vi "Init Agilent Channels Wilt.vi"(0 "Agilent Number":i32, 1 "VISA Resource Name":refnum<visa-resource-name>, 5 "Agilent Channels Array":T1[](array[typedef]), 11 "error in (no error)":errorcluster) -> (4 "Number of Read Channels":i32, 15 "error out":errorcluster)   [LabVIEW 2012]
uses:
  Agilent Channel Definition.ctl
  Drivers/Agilent 34970/Agilent 34970.lvlib
panel:
  out "Channel List":string
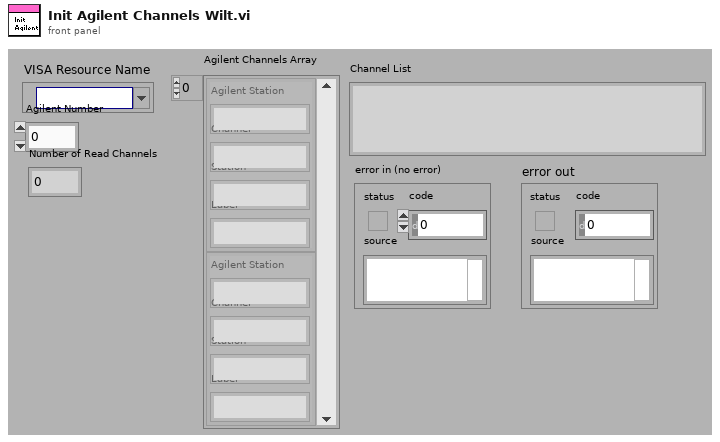
[diagram p1: front panel]
types:
  T1 = typedef "Agilent Channel Definition.ctl" = cluster{"Channel":string, "Station":string, "Label":string, "Agilent Station":string}
  T2 = cluster{"Thermocouple Type (Last)":enum16{"B", "E", "J", "K", "N", "R", "S", "T", "Default (Last)"}, "TC Rjunction (2:Int)":enum16{"Fixed", "External", "Internal"}, "Fixed Rjunction Temp (0:Manual)":enum16{"Manual", "Minimum", "Maximum"}, "TC Auto Check? (F:Don't Check)":bool, "Rjunct Temp Value (0)":dbl}
  T3 = enum16{"100 mV", "1 V", "10 V", "100 V", "300 V", "Minimum", "Maximum"}
  T4 = enum16{"100 Ohm", "1 kOhm", "10 kOhm", "100 kOhm", "1 MOhm", "10 MOhm", "100 MOhm", "Minimum", "Maximum"}
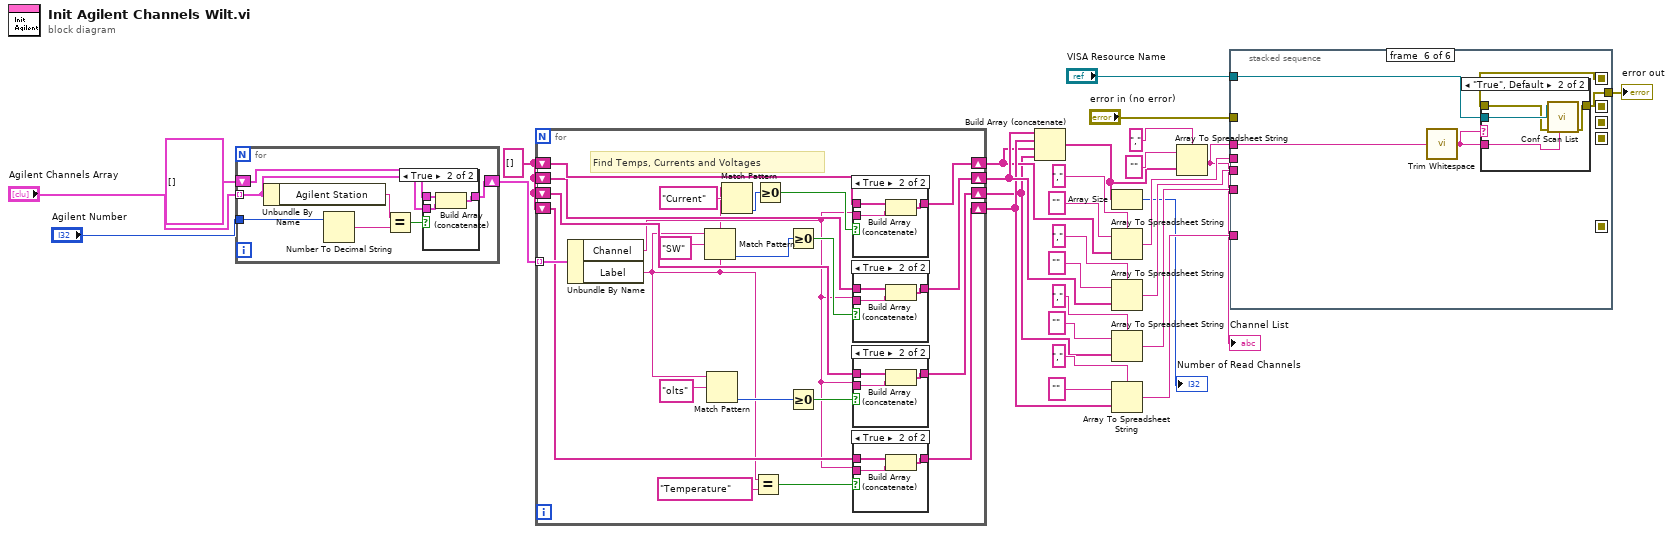
[diagram p0: block diagram]
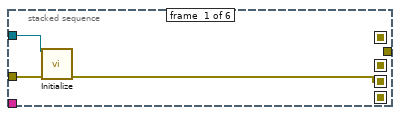
[diagram p3: hidden frame]
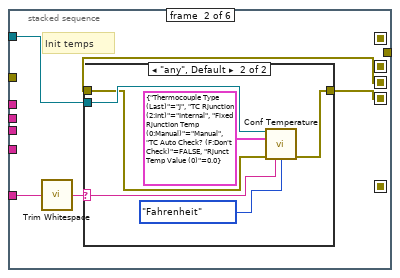
[diagram p4: hidden frame]
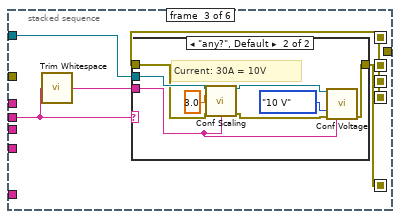
[diagram p6: hidden frame]
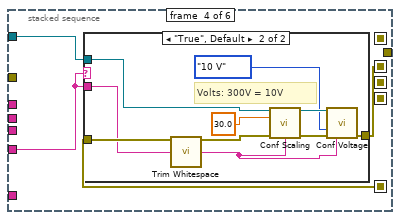
[diagram p8: hidden frame]
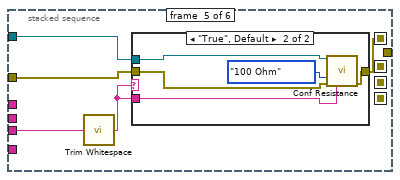
[diagram p10: hidden frame]
diagram:
  w13 = string[] []
  n1 = for {
    tunnel: "Agilent Channels Array" -> [w34] mode=indexing
    tunnel: "Agilent Number" -> [w31]
    shift-right: [w33] -> w14
    shift-left: T1[] [] -> [w32]
    n2 = Unbundle By Name(w34) -> ("Agilent Station"=w35:string)
    n3 = Number To Decimal String(number=w31) -> (decimal integer string=w36:string)  [unwired: 1 in]
    n4 = Equal?(x=w35, y=w36) -> (x = y?=w30:bool)
    n5 = case shown="True" w30 {
      tunnel: w34 -> [_ w40]
      tunnel: [w37 w39] -> w33
      tunnel: w32 -> [w37 w38]
      frame False {
      }
      frame True {
        n6 = Build Array (concatenate)(w38, w40) -> (w39:T1[])
      }
    }
  }
  n7 = for {
    tunnel: w14 -> [w62] mode=indexing
    shift-right: [w59] -> w6
    shift-left: w13 -> [w58]
    shift-right: [w54] -> w5
    shift-left: w13 -> [w53]
    shift-right: [w49] -> w4
    shift-left: w13 -> [w48]
    shift-right: [w44] -> w7
    shift-left: w13 -> [w43]
    # "Find Temps, Currents and Voltages"
    n8 = Unbundle By Name(w62) -> ("Channel"=w42:string, "Label"=w41:string)
    n9 = Match Pattern(string=w41, regular expression="SW") -> (offset past match=w46:i32)  [unwired: 1 in, 3 out]
    n10 = Match Pattern(string=w41, regular expression="olts") -> (offset past match=w51:i32)  [unwired: 1 in, 3 out]
    n11 = Match Pattern(string=w41, regular expression="Current") -> (offset past match=w56:i32)  [unwired: 1 in, 3 out]
    n12 = Equal?(x=w41, y="Temperature") -> (x = y?=w60:bool)
    n13 = Greater Or Equal To 0?(x=w56) -> (x >= 0?=w55:bool)
    n14 = Greater Or Equal To 0?(x=w46) -> (x >= 0?=w47:bool)
    n15 = Greater Or Equal To 0?(x=w51) -> (x >= 0?=w50:bool)
    n16 = case shown="True" w55 {
      tunnel: w42 -> [_ w74]
      tunnel: [w71 w73] -> w54
      tunnel: w53 -> [w71 w72]
      frame False {
      }
      frame True {
        n17 = Build Array (concatenate)(w72, w74) -> (w73:string[])
      }
    }
    n18 = case shown="True" w47 {
      tunnel: w42 -> [_ w66]
      tunnel: [w63 w65] -> w44
      tunnel: w43 -> [w63 w64]
      frame False {
      }
      frame True {
        n19 = Build Array (concatenate)(w64, w66) -> (w65:string[])
      }
    }
    n20 = case shown="True" w50 {
      tunnel: w42 -> [_ w70]
      tunnel: [w67 w69] -> w49
      tunnel: w48 -> [w67 w68]
      frame False {
      }
      frame True {
        n21 = Build Array (concatenate)(w68, w70) -> (w69:string[])
      }
    }
    n22 = case shown="True" w60 {
      tunnel: w42 -> [_ w78]
      tunnel: [w75 w77] -> w59
      tunnel: w58 -> [w75 w76]
      frame False {
      }
      frame True {
        n23 = Build Array (concatenate)(w76, w78) -> (w77:string[])
      }
    }
  }
  n24 = Build Array (concatenate)(w7, w6, w5, w4) -> (w2:string[])
  n25 = Array Size(array=w2) -> (size(s)=→"Number of Read Channels":i32)
  n26 = Array To Spreadsheet String(delimiter (Tab)=",", array=w5, 3:"" ("format string")) -> (spreadsheet string=w22:string)
  n27 = Array To Spreadsheet String(delimiter (Tab)=",", array=w7, 3:"" ("format string")) -> (spreadsheet string=w10:string)
  n28 = Array To Spreadsheet String(delimiter (Tab)=",", array=w4, 3:"" ("format string")) -> (spreadsheet string=w20:string)
  n29 = Array To Spreadsheet String(delimiter (Tab)=",", array=w6, 3:"" ("format string")) -> (spreadsheet string=w27:string)
  n30 = Array To Spreadsheet String(delimiter (Tab)=",", array=w2, 3:"" ("format string")) -> (spreadsheet string=w3:string)
  "Channel List" <- w3
  n31 = stacked-sequence {
    seq-local: [_ _ _ w109 _ _] -> [_ _ _ _ _ _]
    seq-local: [_ _ w96 _ _ _] -> [_ _ _ w110 _ _]
    seq-local: [_ w85 _ _ _ _] -> [_ _ w97 _ _ _]
    seq-local: [w80 _ _ _ _ _] -> [_ w84 _ _ _ _]
    seq-local: [_ _ _ _ w124 _] -> [_ _ _ _ _ w135]
    tunnel: w27 -> [_ w83 _ _ _ _]
    tunnel: "VISA Resource Name" -> [w79 w86 w98 w111 w125 w137]
    tunnel: w22 -> [_ _ w94 _ _ _]
    tunnel: w20 -> [_ _ _ w108 _ _]
    tunnel: "error in (no error)" -> [w81 _ _ _ w126 _]
    tunnel: [_ _ _ _ _ w136] -> w18
    tunnel: w10 -> [_ _ _ _ w123 _]
    tunnel: w3 -> [_ _ _ _ _ w134]
    frame #0 {
      n32 = call "Initialize.vi"("VISA Resource Name"=w79, "error in (no error)"=w81) -> ("error out"=w80:errorcluster)  [unwired: 12 in, 1 out]
    }
    frame #1 {
      # "Init temps"
      n33 = call <vilib>:"Trim Whitespace.vi"("string"=w83) -> ("trimmed string"=w82:string)  [unwired: 1 in]
      n34 = case shown="\"any\", Default" w82 {
        selector: w82 -> [_ w88]
        tunnel: w86 -> [_ w91]
        tunnel: [w87 w90] -> w85
        tunnel: w84 -> [w87 w89]
        frame "" {
        }
        frame "any", Default {
          n35 = call "Conf Temperature.vi"("VISA Resource Name"=w91, "Thermocouple Configuration"=T2 {"Thermocouple Type (Last)"=enum."J", "TC Rjunction (2:Int)"=enum."Internal", "Fixed Rjunction Temp (0:Manual)"=enum."Manual", "TC Auto Check? (F:Don't Check)"=FALSE, "Rjunct Temp Value (0)"=0.0}, "error in (no error)"=w89, "Channel List(empty)"=w88, "Units (0:Celsius)"=enum16{"Celsius", "Fahrenheit", "Kelvin"}."Fahrenheit") -> ("error out"=w90:errorcluster)  [unwired: 8 in, 2 out]
        }
      }
    }
    frame #2 {
      n36 = call <vilib>:"Trim Whitespace.vi"("string"=w94) -> ("trimmed string"=w95:string)  [unwired: 1 in]
      n37 = case shown="\"any?\", Default" w94 {
        tunnel: w98 -> [_ w107]
        tunnel: w97 -> [w99 w102]
        tunnel: [w99 w101] -> w96
        tunnel: w95 -> [_ w100]
        frame "" {
        }
        frame "any?", Default {
          # "Current: 30A = 10V"
          n38 = call "Conf Scaling.vi"("VISA Resource Name"=w107, "Gain (1)"=3.0, "error in (no error)"=w102, "Channel List (empty)"=w100) -> ("VISA Resource Name Out"=w106:refnum<visa-resource-name>, "error out"=w105:errorcluster)  [unwired: 9 in, 1 out]
          n39 = call "Conf Voltage.vi"("VISA Resource Name"=w106, "Range (6:Max)"=T3."10 V", "error in (no error)"=w105, "Channel List (empty)"=w100) -> ("error out"=w101:errorcluster)  [unwired: 9 in, 2 out]
        }
      }
    }
    frame #3 {
      n40 = case shown="\"True\", Default" w108 {
        tunnel: w111 -> [_ w121]
        tunnel: w110 -> [w112 w116]
        tunnel: [w112 w115] -> w109
        tunnel: w108 -> [_ w114]
        frame "" {
        }
        frame "True", Default {
          # "Volts: 300V = 10V"
          n41 = call <vilib>:"Trim Whitespace.vi"("string"=w114) -> ("trimmed string"=w113:string)  [unwired: 1 in]
          n42 = call "Conf Scaling.vi"("VISA Resource Name"=w121, "Gain (1)"=30.0, "error in (no error)"=w116, "Channel List (empty)"=w113) -> ("VISA Resource Name Out"=w120:refnum<visa-resource-name>, "error out"=w119:errorcluster)  [unwired: 9 in, 1 out]
          n43 = call "Conf Voltage.vi"("VISA Resource Name"=w120, "Range (6:Max)"=T3."10 V", "error in (no error)"=w119, "Channel List (empty)"=w113) -> ("error out"=w115:errorcluster)  [unwired: 9 in, 2 out]
        }
      }
    }
    frame #4 {
      n44 = call <vilib>:"Trim Whitespace.vi"("string"=w123) -> ("trimmed string"=w122:string)  [unwired: 1 in]
      n45 = case shown="\"True\", Default" w122 {
        tunnel: w126 -> [w127 w132]
        tunnel: w125 -> [_ w131]
        tunnel: [w127 w130] -> w124
        tunnel: w122 -> [_ w129]
        frame "" {
        }
        frame "True", Default {
          n46 = call "Conf Resistance.vi"("VISA Resource Name"=w131, "Range (8:Maximum)"=T4."100 Ohm", "error in (no error)"=w132, "Channel List (empty)"=w129) -> ("error out"=w130:errorcluster)  [unwired: 9 in, 2 out]
        }
      }
    }
    frame #5 {
      n47 = call <vilib>:"Trim Whitespace.vi"("string"=w134) -> ("trimmed string"=w133:string)  [unwired: 1 in]
      n48 = case shown="\"True\", Default" w133 {
        tunnel: w137 -> [_ w142]
        tunnel: [w138 w141] -> w136
        tunnel: w135 -> [w138 w140]
        tunnel: w133 -> [_ w139]
        frame "" {
        }
        frame "True", Default {
          n49 = call "Conf Scan List.vi"("Scan List (empty)"=w139, "error in (no error)"=w140, "VISA Resource Name"=w142) -> ("error out"=w141:errorcluster)  [unwired: 6 in, 2 out]
        }
      }
    }
  }
  "error out" <- w18
